vi "Sort String Array By Length.vi"(8 "Order (descending)":enum16{"ascending", "descending"}(ring)=enum."descending", 11 "String Array":string[](array[string])) -> (0 "Sorted Pointers":i32[](array[numeric]), 3 "Sorted String Array":string[](array[string]))   [LabVIEW 2021, in "Strings.lvlib"]
uses:
  <userlib>/_OpenG.lib/array/array.llb/Sort 1D Array (I32)__ogtk.vi
  <userlib>/_OpenG.lib/array/array.llb/Reorder 1D Array2 (String)__ogtk.vi
  Strings.lvlib
  <userlib>/_OpenG.lib/array/array.llb/openg_array.lvlib
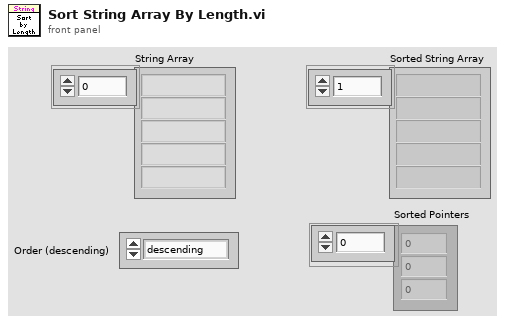
[diagram p1: front panel]
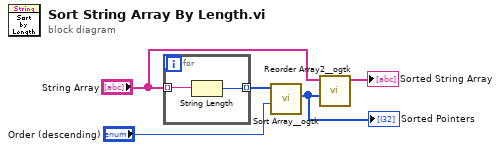
[diagram p0: block diagram]
diagram:
  n1 = for {
    tunnel: "String Array" -> [w7] mode=indexing
    tunnel: [w6] -> w5 mode=indexing
    n2 = String Length(string=w7) -> (length=w6:i32)
  }
  n3 = call-poly <userlib>:"Sort Array__ogtk.vi"("Order"="Order (descending)", "Array in"=w5) -> ("Sorted Pointers"=w4:i32[])  [unwired: 8 in, 1 out]
  "Sorted Pointers" <- w4
  n4 = call-poly <userlib>:"Reorder Array2__ogtk.vi"("indices"=w4, "array"="String Array") -> ("reordered array"=→"Sorted String Array":string[])  [unwired: 9 in]
